vi "Send Pre-Addressed Unsubscribe.vi"(8 "error in (no error)":errorcluster, 10 "SubscriptionPolicy":T1, 11 "Unsubscribe Msg In":refnum<class "Unsubscribe Msg.lvclass">) -> (0 "error out":errorcluster)   [LabVIEW 2017, in "IMediator.lvlib" / "Unsubscribe Msg.lvclass"]
doc: "Most Actors or VIs that want to publish data will do so with this send VI. Actors who call this method must have been given a pre-addressed Publish Msg prior to the act of sending. (For Actors, this means that they were launched with a pre-addressed Publish Msg or sent one after the Mediator came alive.)\n\n<License>\nCopyright © 2017 Composed Systems, LLC | All rights reserved\nwww.composed.io\n\nAuthor: Ethan Stern <ethan.stern@composed.io>\n\nThis software is provided \"AS IS\" WITHOUT WARRANTIES, either express or implied, AND IS FOR EDUCATIONAL PURPOSES ONLY.\n</License>"
uses:
  Unsubscribe Msg.lvclass
  C:/Git/mva-framework/Framework/AbstractMessages/PreAddressedMsg/PreAddressedMsg.lvclass
  C:/Program Files (x86)/National Instruments/LabVIEW 2017/vi.lib/ActorFramework/Message/Message.lvclass
  ISubscriptionPolicy/ISubscriptionPolicy Reference.ctl
  ISubscriptionPolicy/ISubscriptionPolicy.lvclass
  AbstractMessages/PreAddressedMsg/PreAddressedMsg.lvclass/PreAddressedMsg.ctl
  Unsubscribe Msg.lvclass/Unsubscribe Msg.ctl
  <vilib>/ActorFramework/Message Enqueuer/Message Enqueuer.lvclass/Message Enqueuer.ctl
  <vilib>/ActorFramework/Message Priority Queue/Priority Enqueue.vi
  <vilib>/ActorFramework/Message Enqueuer/Message Enqueuer.lvclass
  AbstractMessages/PreAddressedMsg/PreAddressedMsg.lvclass
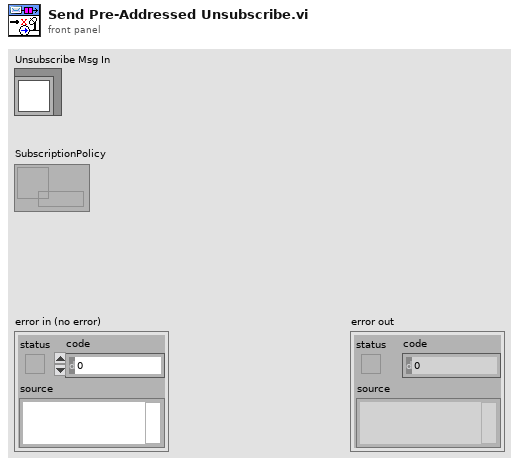
[diagram p1: front panel]
types:
  T1 = typedef "IMediator.lvlib/ISubscriptionPolicy.lvclass/ISubscriptionPolicy Reference.ctl" = refnum<data-value>
  T2 = typedef "Actor Framework.lvlib/Message Enqueuer.lvclass/Message Priority.ctl" = enum16{"Low", "Normal", "High"}
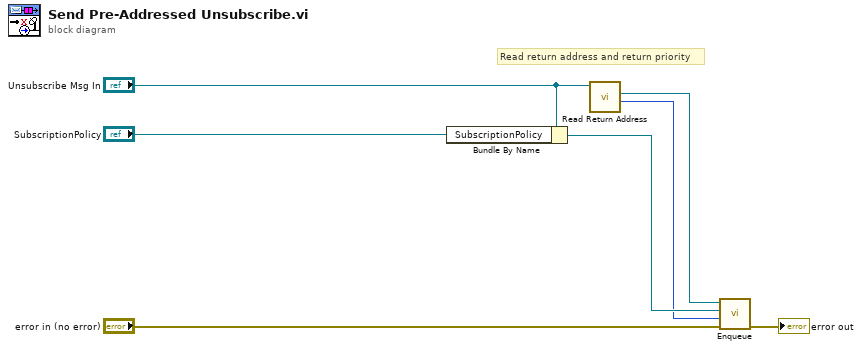
[diagram p0: block diagram]
diagram:
  # "Read return address and return priority"
  n1 = Bundle By Name(cluster="Unsubscribe Msg In", "SubscriptionPolicy"="SubscriptionPolicy") -> (w5:refnum<class "Unsubscribe Msg.lvclass">)
  n2 = call "Read Return Address.vi"("PreAddressedMsg in"="Unsubscribe Msg In") -> ("Return Priority (Normal)"=w3:T2, "Return Address"=w4:refnum<class "Message Enqueuer.lvclass">)  [unwired: 9 in]
  n3 = call <vilib>:"Enqueue.vi"("error in (no error)"="error in (no error)", "Message Priority (Normal)"=w3, "Message"=w5, "Message Enqueuer in"=w4) -> ("error out"=→"error out":errorcluster)  [unwired: 6 in, 1 out]
